vi "日報表New.vi"(9 "End Date":string="2014/11/13") -> (0 "error out 2":errorcluster)   [LabVIEW 2012]
uses:
  <vilib>/Utility/NIReport.llb/NI_report.lvclass
  Global1.vi
  <vilib>/Utility/NIReport.llb/Append Text Table to Report (wrap).vi
  <vilib>/Utility/NIReport.llb/Excel/NI_Excel.lvclass
  <vilib>/addons/_office/NI_ReportGenerationToolkit.lvlib
panel:
  out "error out":errorcluster
  in  "ShiftB":string[][](array[string])
  in  "ShiftA":string[][](array[string])
  in  "ShiftC":string[][](array[string])
  in  "Summary":string[][](array[string])
  out "Row Headers":string[](array[string])
  in  "MonthToDate":string[][](array[string])
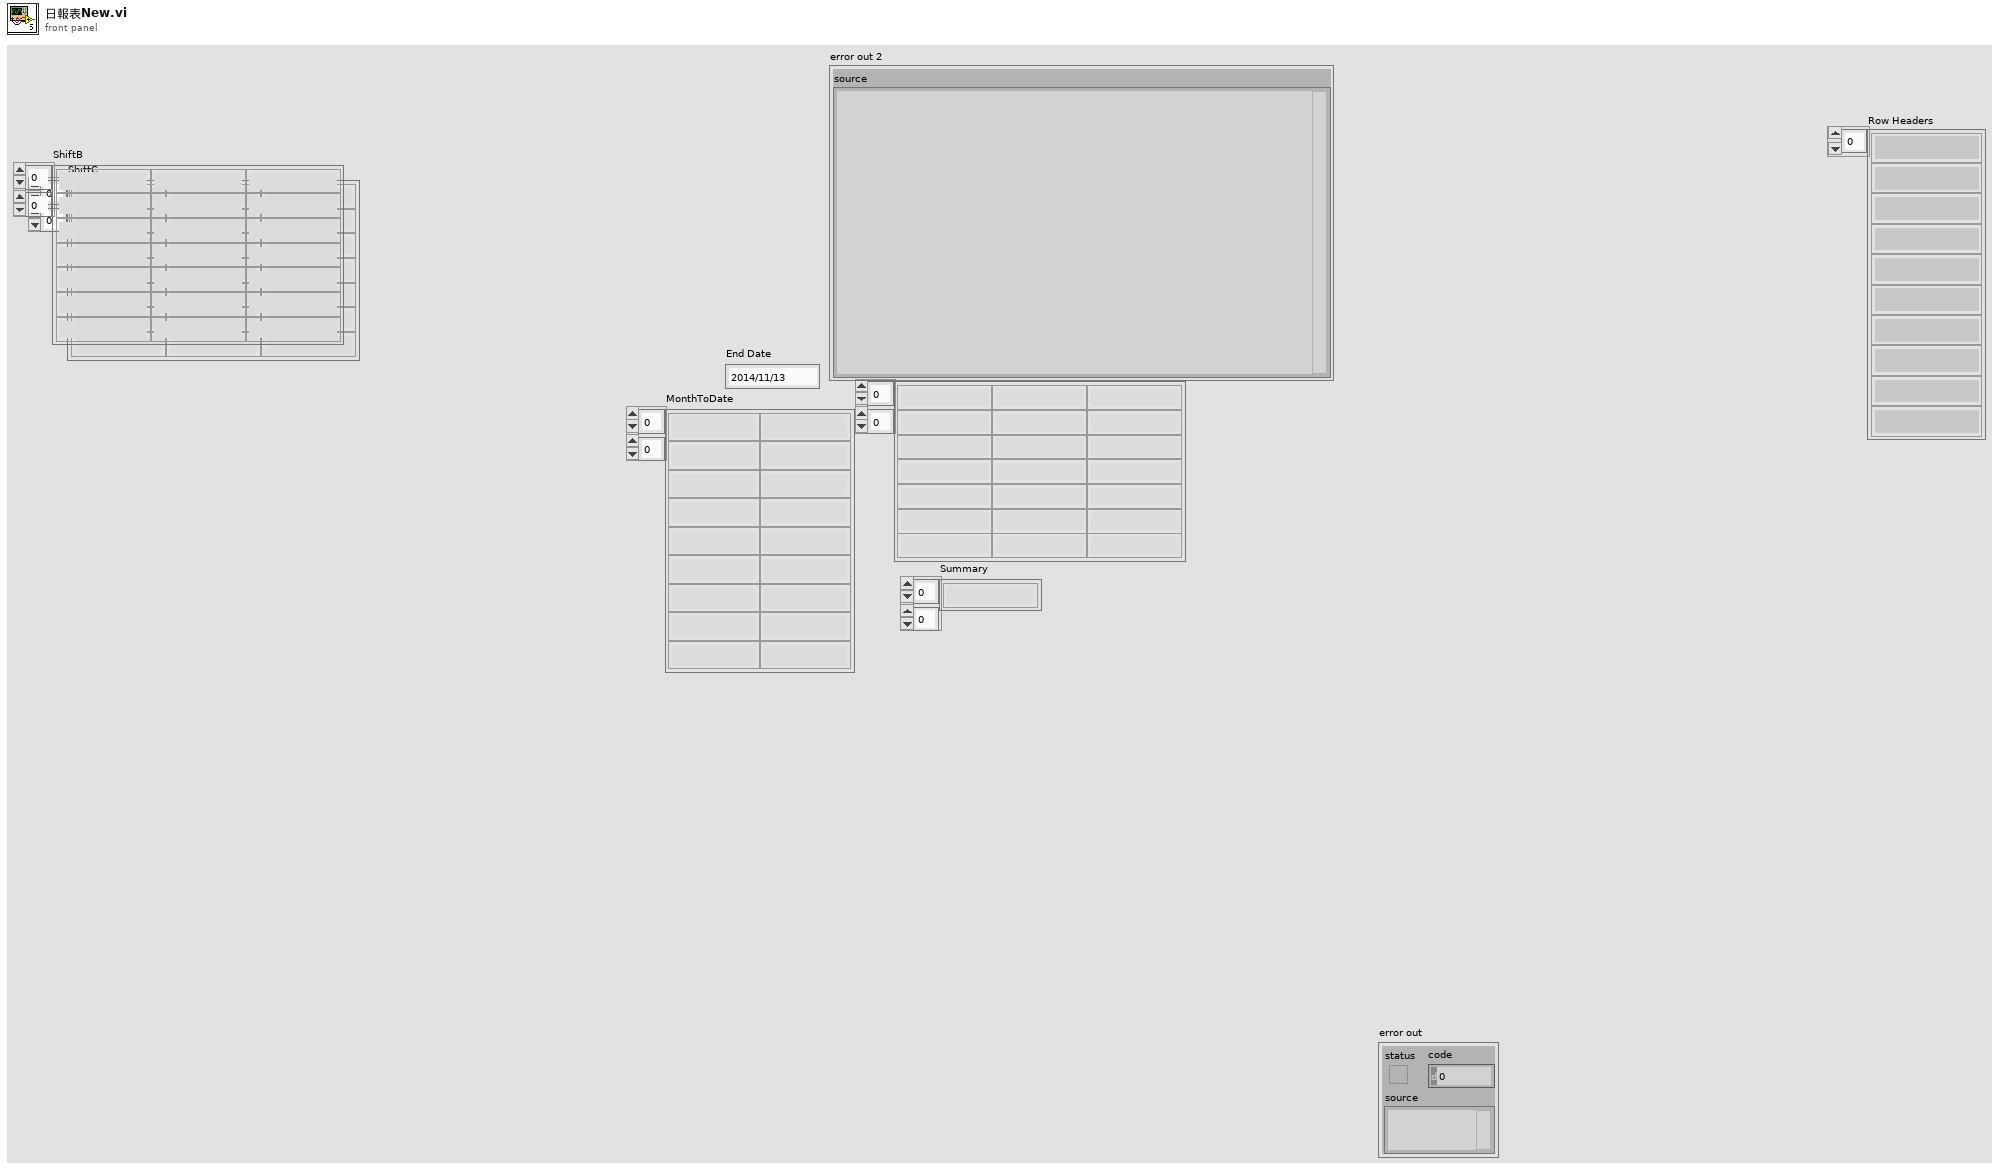
[diagram p1: front panel]
types:
  T1 = enum16{"Standard Report", "HTML", "Word", "Excel"}
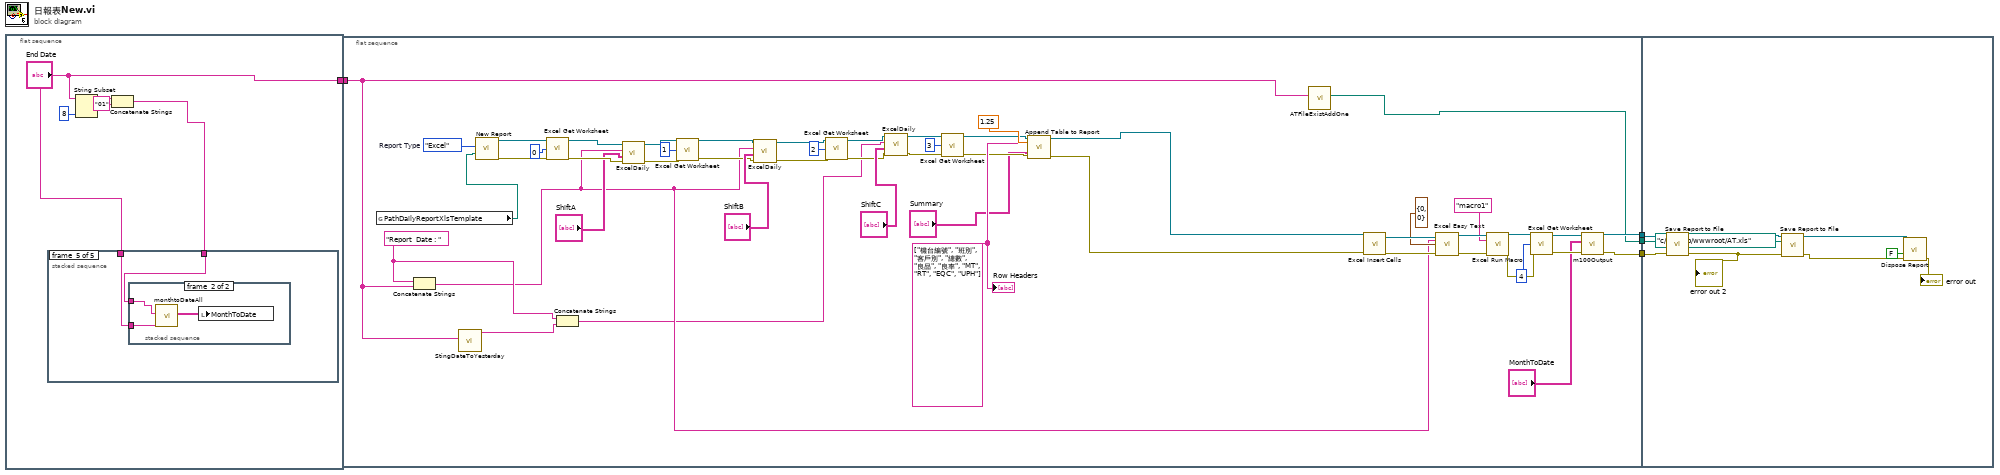
[diagram p0: block diagram]
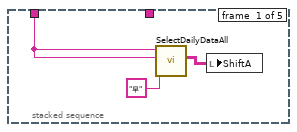
[diagram p2: hidden frame]
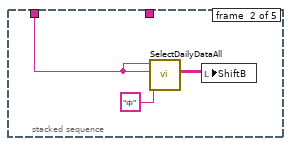
[diagram p3: hidden frame]
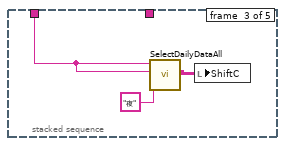
[diagram p4: hidden frame]
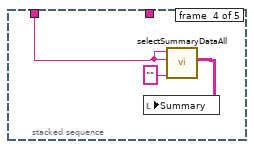
[diagram p5: hidden frame]
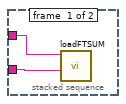
[diagram p6: hidden frame]
diagram:
  n1 = flat-sequence {
    tunnel: ["End Date"] -> w1
    frame #0 {
      n2 = String Subset(string="End Date", length (rest)=8 ("length (rest)")) -> (substring=w8:string)  [unwired: 1 in]
      n3 = Concatenate Strings(w8, "01" ("string")) -> (w6:string)
      n4 = stacked-sequence {
        tunnel: w6 -> [_ _ _ _ w22]
        tunnel: "End Date" -> [w10 w13 w16 w19 w23]
        frame #0 {
          n5 = call "SelectDailyDataAll.vi"("Shift"="早", "End_date"=w10, "Begin_date"=w10) -> ("output array"=w11:string[][])  [unwired: 8 in]
          n6 = local write "ShiftA"(w11) -> ()
        }
        frame #1 {
          n7 = call "SelectDailyDataAll.vi"("Shift"="中", "End_date"=w13, "Begin_date"=w13) -> ("output array"=w14:string[][])  [unwired: 8 in]
          n8 = local write "ShiftB"(w14) -> ()
        }
        frame #2 {
          n9 = call "SelectDailyDataAll.vi"("Shift"="夜", "End_date"=w16, "Begin_date"=w16) -> ("output array"=w17:string[][])  [unwired: 8 in]
          n10 = local write "ShiftC"(w17) -> ()
        }
        frame #3 {
          n11 = call "selectSummaryDataAll.vi"("Shift"="", "End_date"=w19, "Begin_date"=w19) -> ("Summary"=w21:string[][])  [unwired: 8 in]
          n12 = local write "Summary"(w21) -> ()
        }
        frame #4 {
          n13 = stacked-sequence {
            tunnel: w23 -> [w25 w26]
            tunnel: w22 -> [w24 w27]
            frame #0 {
              n14 = call "loadFTSUM.vi"("End Date"=w25, "From Date"=w24) -> ()  [unwired: 9 in, 1 out]
            }
            frame #1 {
              n15 = call "monthtoDateAll.vi"("End Date"=w26, "From Date"=w27) -> ("output array"=w28:string[][])  [unwired: 8 in, 1 out]
              n16 = local write "MonthToDate"(w28) -> ()
            }
          }
        }
      }
    }
  }
  n17 = flat-sequence {
    tunnel: w1 -> [w35]
    tunnel: [w38] -> w4
    tunnel: [w37] -> w3
    tunnel: [w36] -> w2
    tunnel: w4 -> [w88]
    tunnel: w3 -> [w87]
    tunnel: w2 -> [w86]
    frame #0 {
      w33 = "Report  Date : " ("string")
      w55 = string[] ["機台編號", "班別", "客戶別", "總數", "良品", "良率", "MT", "RT", "EQC", "UPH"] ("row headers")
      w78 = T1."Excel"  # Report Type
      n18 = global read "Global1.vi" "PathDailyReportXlsTemplate"() -> (w39:path)
      n19 = Concatenate Strings(w33, w35) -> (w32:string)
      n20 = call "StingDateToYesterday.vi"("Date"=w35) -> ("Date+1"=w34:string)  [unwired: 9 in, 1 out]
      n21 = call <vilib>:"New Report.vi"("report type"=w78, "template (empty)"=w39) -> ("report out"=w77:refnum<class "NI_report.lvclass">, "error out"=w76:errorcluster)  [unwired: 12 in]
      n22 = call <vilib>:"Excel Get Worksheet.vi"("report in"=w77, "worksheet index (0)"=0, "error in (no error)"=w76) -> ("report out"=w74:refnum<class "NI_report.lvclass">, "error out"=w73:errorcluster)  [unwired: 11 in]
      n23 = Concatenate Strings(w33, w34) -> (w31:string)
      n24 = call "ExcelDaily.vi"("error in (no error)"=w73, "Input"="ShiftA", "Header"=w32, "report in"=w74) -> ("error out"=w67:errorcluster, "report out"=w69:refnum<class "NI_report.lvclass">)  [unwired: 6 in]
      n25 = call <vilib>:"Excel Get Worksheet.vi"("report in"=w69, "worksheet index (0)"=1, "error in (no error)"=w67) -> ("report out"=w68:refnum<class "NI_report.lvclass">, "error out"=w66:errorcluster)  [unwired: 11 in]
      n26 = call "ExcelDaily.vi"("error in (no error)"=w66, "Input"="ShiftB", "Header"=w32, "report in"=w68) -> ("error out"=w63:errorcluster, "report out"=w64:refnum<class "NI_report.lvclass">)  [unwired: 6 in]
      n27 = call <vilib>:"Excel Get Worksheet.vi"("report in"=w64, "worksheet index (0)"=2, "error in (no error)"=w63) -> ("report out"=w62:refnum<class "NI_report.lvclass">, "error out"=w61:errorcluster)  [unwired: 11 in]
      n28 = call "ExcelDaily.vi"("error in (no error)"=w61, "Input"="ShiftC", "Header"=w31, "report in"=w62) -> ("error out"=w58:errorcluster, "report out"=w59:refnum<class "NI_report.lvclass">)  [unwired: 6 in]
      n29 = call <vilib>:"Excel Get Worksheet.vi"("report in"=w59, "worksheet index (0)"=3, "error in (no error)"=w58) -> ("report out"=w48:refnum<class "NI_report.lvclass">, "error out"=w47:errorcluster)  [unwired: 11 in]
      n30 = call-poly <vilib>:"Append Table to Report.vi"("report in"=w48, "column width (1)"=1.25, "column headers"=w55, "text data"="Summary", "error in (no error)"=w47) -> ("report out"=w30:refnum<class "NI_report.lvclass">, "error out"=w29:errorcluster)  [unwired: 7 in, 2 out]
      n31 = call "ATFileExistAddOne.vi"("input string"=w35) -> ("appended path"=w36:path)  [unwired: 10 in]
      n32 = call <vilib>:"Excel Insert Cells.vi"("report in"=w30, "error in (no error)"=w29) -> ("report out"=w54:refnum<class "NI_report.lvclass">, "error out"=w53:errorcluster)  [unwired: 12 in]
      n33 = call <vilib>:"Excel Easy Text.vi"("report in"=w54, "text"=w32, "start (-1, -1)"=cluster{"row":i32, "column":i32} {"row"=0, "column"=0} ("end (-1, -1)"), "error in (no error)"=w53) -> ("report out"=w51:refnum<class "NI_report.lvclass">, "error out"=w50:errorcluster)  [unwired: 7 in, 3 out]
      n34 = call <vilib>:"Excel Run Macro.vi"("report in"=w51, "macro name"="macro1", "error in (no error)"=w50) -> ("report out"=w45:refnum<class "NI_report.lvclass">, "error out"=w44:errorcluster)  [unwired: 10 in, 1 out]
      n35 = call <vilib>:"Excel Get Worksheet.vi"("report in"=w45, "worksheet index (0)"=4, "error in (no error)"=w44) -> ("report out"=w42:refnum<class "NI_report.lvclass">, "error out"=w41:errorcluster)  [unwired: 11 in]
      n36 = call "m100Output.vi"("error in (no error)"=w41, "Input"="MonthToDate", "report in"=w42) -> ("error out"=w37:errorcluster, "report out"=w38:refnum<class "NI_report.lvclass">)  [unwired: 7 in]
      "Row Headers" <- w55
    }
    frame #1 {
      n37 = call-dynamic "Save Report to File.vi"("report in"=w88, "report file path"=w86, "error in (no error)"=w87) -> ("report out"=w83:refnum<class "NI_report.lvclass">, "error out"=w81:errorcluster)  [unwired: 11 in]
      "error out 2" <- w81
      n38 = call-dynamic "Save Report to File.vi"("report in"=w83, "report file path"=path "c:/inetpub/wwwroot/AT.xls", "error in (no error)"=w81) -> ("report out"=w82:refnum<class "NI_report.lvclass">, "error out"=w80:errorcluster)  [unwired: 11 in]
      n39 = call-dynamic "Dispose Report.vi"("report in"=w82, "save changes? (F)"=FALSE, "error in (no error)"=w80) -> ("error out"=→"error out":errorcluster)  [unwired: 12 in]
    }
  }
